vi "TitleBar.CreateRequests.vi"(8 "error in (no error)":errorcluster) -> (0 "error out":errorcluster, 3 "Requests":T1)   [LabVIEW 2024, in "TitleBar.lvclass"]
uses:
  TitleBar.lvclass
  Request Events--cluster.ctl
  Do Something Args.ctl
  JQMHCore/Module/Reply.ctl
  AddTopLevelVI Args.ctl
  TitleBar.lvclass/TitleBar.ctl
  JQMHCore/Module/RQMHModule.lvclass
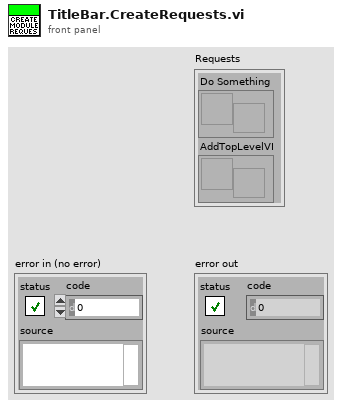
[diagram p1: front panel]
types:
  T1 = typedef "TitleBar.lvclass/Request Events--cluster.ctl" = cluster{"Do Something":refnum<user-event>, "AddTopLevelVI":refnum<user-event>}
  T2 = typedef "TitleBar.lvclass/AddTopLevelVI Args.ctl" = cluster{"MainRef":refnum<vi>}
  T3 = typedef "RQMHModule.lvclass/Reply.ctl" = cluster{"Expects Reply":bool, "Reply":refnum<notifier>}
  T4 = cluster{"AddTopLevelVI Args":T2, "Reply Payload":T3}
  T5 = typedef "TitleBar.lvclass/Do Something Args.ctl" = cluster{"Msg":string}
  T6 = cluster{"Do Something Args":T5, "Reply Payload":T3}
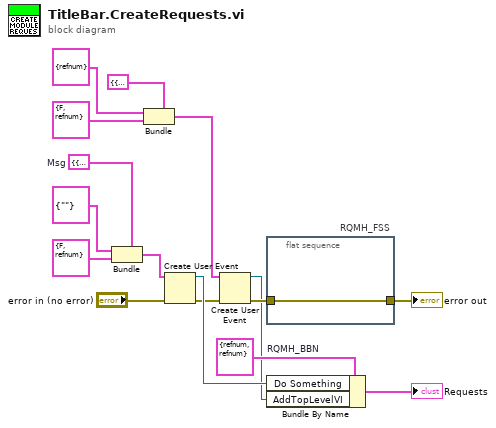
[diagram p0: block diagram]
diagram:
  w10 = T6 {"Do Something Args"={"Msg"=""}, "Reply Payload"={"Expects Reply"=FALSE, "Reply"=refnum}}  # Msg
  n1 = Bundle(cluster=w10, "Do Something Args"=T5 {"Msg"=""}, "Reply Payload"=T3 {"Expects Reply"=FALSE, "Reply"=refnum}) -> (w13:T6)
  n2 = Bundle(cluster=T4 {"AddTopLevelVI Args"={"MainRef"=refnum}, "Reply Payload"={"Expects Reply"=FALSE, "Reply"=refnum}}, "AddTopLevelVI Args"=T2 {"MainRef"=refnum}, "Reply Payload"=T3 {"Expects Reply"=FALSE, "Reply"=refnum}) -> (w2:T4)
  n3 = Create User Event(user event datatype=w13, error in="error in (no error)") -> (user event=w9:refnum<user-event>, error out=w4:errorcluster)
  n4 = Create User Event(user event datatype=w2, error in=w4) -> (user event=w1:refnum<user-event>, error out=w3:errorcluster)
  n5 = flat-sequence "RQMH_FSS" {
    tunnel: [w17] -> w8
    tunnel: w3 -> [w17]
    frame #0 {
    }
  }
  n6 = Bundle By Name "RQMH_BBN"(cluster=T1 {"Do Something"=refnum, "AddTopLevelVI"=refnum} ("Requests"), "Do Something"=w9, "AddTopLevelVI"=w1) -> (→"Requests":T1)
  "error out" <- w8
